vi "read pre and post build refs .vi"(11 "Builders in":refnum<class "Builder.lvclass">) -> (2 "pre and post build refs":refnum<vi>[](array[refnum]))   [LabVIEW 2024, in "Builder.lvclass"]
uses:
  Builder.lvclass
  Builder.lvclass/Builder.ctl
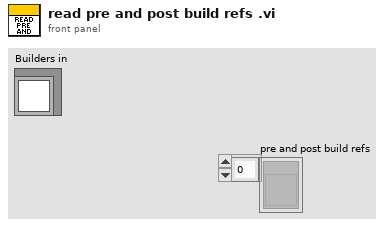
[diagram p1: front panel]
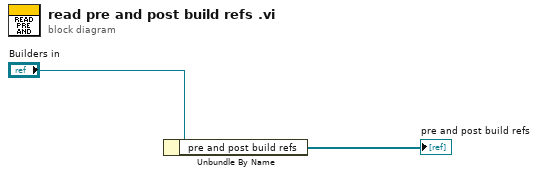
[diagram p0: block diagram]
diagram:
  n1 = Unbundle By Name("Builders in") -> ("pre and post build refs"=→"pre and post build refs":refnum<vi>[])
